vi "Deploy ABORT.vi"   [LabVIEW 2020]
uses:
  <vilib>/lvdsc/process/Deploy Library.vi
  <vilib>/lvdsc/NI_DSC.lvlib
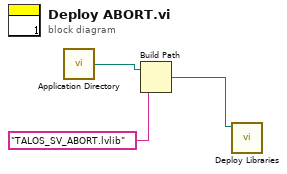
[diagram p0: block diagram]
diagram:
  n1 = call <vilib>:"Application Directory.vi"() -> ("Application Directory"=w3:path)
  n2 = Build Path(base path=w3, name or relative path="TALOS_SV_ABORT.lvlib") -> (appended path=w1:path)
  n3 = call-poly <vilib>:"Deploy Libraries.vi"("library path"=w1) -> ()  [unwired: 8 in, 1 out]
